vi "Write X.vi"(8 "error in (no error)":errorcluster, 10 "X":waveform(dbl)[](array[waveform]), 11 "DSP in":refnum<class "DSP.lvclass">) -> (0 "error out":errorcluster, 3 "DSP out":refnum<class "DSP.lvclass">)   [LabVIEW 2019, in "DSP.lvclass"]
uses:
  DSP.lvclass
  DSP.lvclass/DSP.ctl
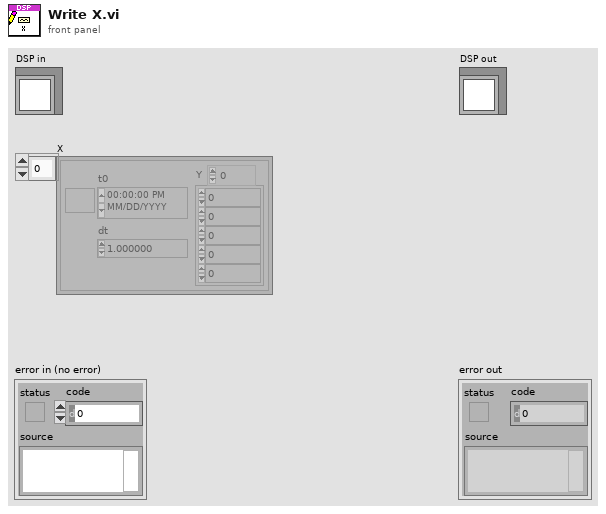
[diagram p1: front panel]
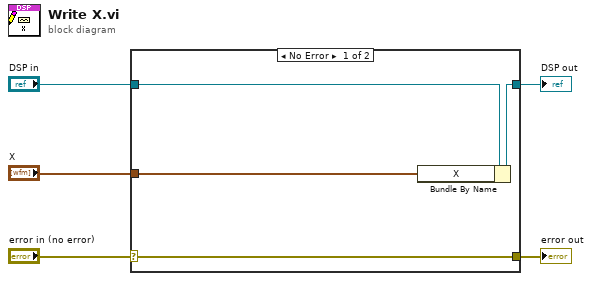
[diagram p0: block diagram]
diagram:
  n1 = case shown="No Error" "error in (no error)" {
    selector: "error in (no error)" -> [w9 w10]
    tunnel: [w9 w10] -> w4
    tunnel: [w7 w11] -> w2
    tunnel: "DSP in" -> [w8 w11]
    tunnel: "X" -> [w6 _]
    frame No Error {
      n2 = Bundle By Name(cluster=w8, "X"=w6) -> (w7:refnum<class "DSP.lvclass">)
    }
    frame Error {
    }
  }
  "error out" <- w4
  "DSP out" <- w2
